vi "Setpoint Angle Global Variable.vi"(10 "Angle":dbl, 11 "T (Set) F (Get":bool) -> (3 "Setpoint Angle":dbl format="%#_13g")   [LabVIEW 2017]
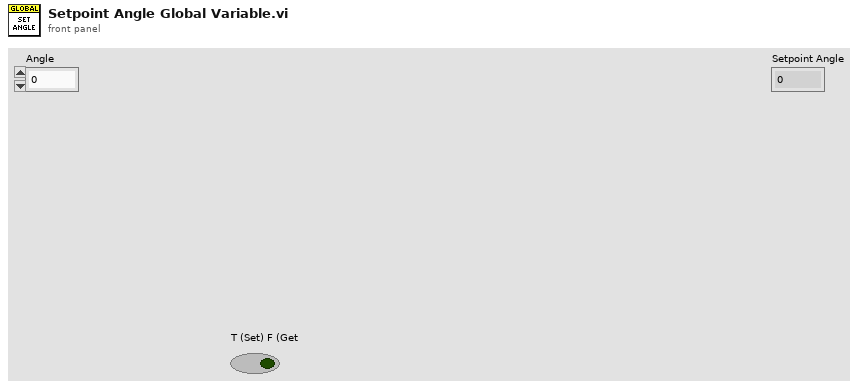
[diagram p1: front panel]
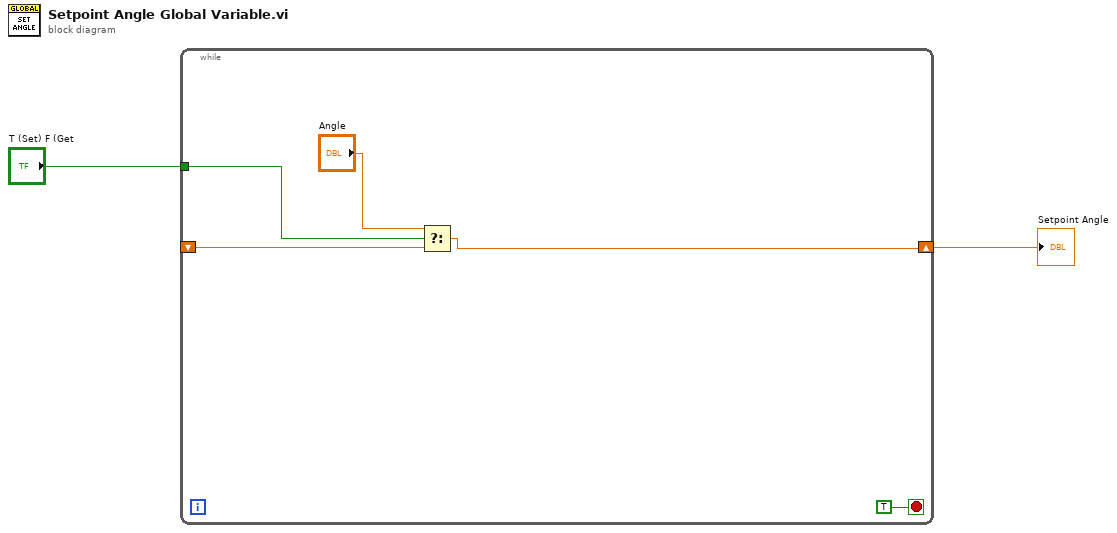
[diagram p0: block diagram]
diagram:
  n1 = while {
    shift-right: [w4] -> w1
    shift-left: _ -> [w5]
    tunnel: "T (Set) F (Get" -> [w6]
    stop <- TRUE stop-if-true
    n2 = Select(t="Angle", s=w6, f=w5) -> (s? t:f=w4:dbl)
  }
  "Setpoint Angle" <- w1
